vi "Dual Image Threshold [U16].vi"(8 "error in (no error)":errorcluster, 9 "Range":cluster{"Lower value":sgl, "Upper value":sgl}={"Lower value"=128.0, "Upper value"=255.0} {"Upper value" format="%.2f"; "Lower value" format="%.2f"}, 10 "Image Dst":T1, 11 "Image Src":T1) -> (0 "error out":errorcluster, 1 "CPU (s)":dbl, 3 "Image Dst Out":T1)   [LabVIEW 2021]
uses:
  <vilib>/vision/Image Controls.llb/IMAQ Image.ctl
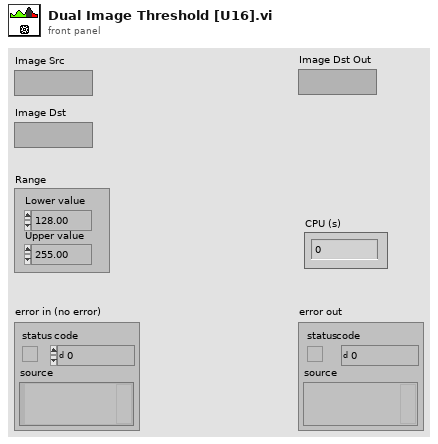
[diagram p1: front panel]
types:
  T1 = typedef "IMAQ Image.ctl" = refnum<image>
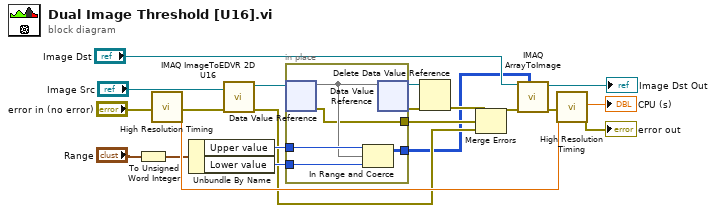
[diagram p0: block diagram]
diagram:
  n1 = To Unsigned Word Integer(number="Range") -> (unsigned 16bit integer=w2:cluster{"Lower value":u16, "Upper value":u16})
  n2 = call "High Resolution Timing.vi"("Error In"="error in (no error)") -> ("elapsed (relative) seconds"=w8:dbl, "Error Out"=w13:errorcluster)  [unwired: 16 in, 1 out]
  n3 = Unbundle By Name(w2) -> ("Upper value"=w18:u16, "Lower value"=w17:u16)
  n4 = call <vilib>:"IMAQ ImageToEDVR 2D U16.vi"("error out"=w13, "Image"="Image Src") -> ("error out"=w3:errorcluster, "EDVR 2D U16"=w20:refnum<data-value>)  [unwired: 7 in, 1 out]
  n5 = in-place {
    in-place-border: w18 -> [w26]
    in-place-border: w17 -> [w24]
    in-place-border: [w25] -> w1
    in-place-border: [w22] -> w6
    n6 = in-place-dvr #1(w20) -> (w23:u16[][], w22:errorcluster)
    n7 = In Range and Coerce(upper limit=w26, x=w23, lower limit=w24) -> (coerced(x)=w25:u16[][])  [unwired: 1 out]
    n8 = in-place-dvr #1(w23) -> (w16:refnum<data-value>, w15:errorcluster)
  }
  n9 = Delete Data Value Reference(data value reference=w16, error in=w15) -> (error out=w4:errorcluster)  [unwired: 1 out]
  n10 = Merge Errors(w4, w6, w3) -> (w5:errorcluster)
  n11 = call "IMAQ ArrayToImage"("Image Pixels (U16)"=w1, "error in (no error)"=w5, "Image"="Image Dst") -> ("error out"=w12:errorcluster, "Image Out"=→"Image Dst Out":T1)  [unwired: 7 in]
  n12 = call "High Resolution Timing.vi"("relative seconds (NaN)"=w8, "Error In"=w12) -> ("elapsed (relative) seconds"=→"CPU (s)":dbl, "Error Out"=→"error out":errorcluster)  [unwired: 15 in, 1 out]
